vi "wd_replaceInIndexFindNext.vi"(9 "Next in":i32, 10 "LengthIn":u64, 11 "RecordInfo":T1[](array[typedef])) -> (2 "LengthOut":u64, 3 "Next out":i32)   [LabVIEW 2020, in "NI_ExcelFile.lvlib"]
uses:
  <vilib>/express/express shared/NI_ExcelFile/NI_ExcelFile.lvlib
  <vilib>/express/express shared/NI_ExcelFile/Ctrls/wd_recordInfo.ctl
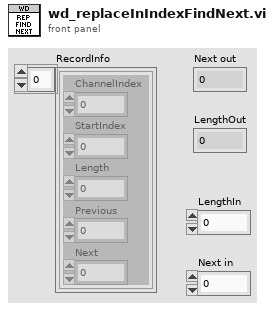
[diagram p1: front panel]
types:
  T1 = typedef "NI_ExcelFile.lvlib/wd_recordInfo.ctl" = cluster{"ChannelIndex":u32, "StartIndex":u64, "Length":u64, "Previous":i32, "Next":i32}
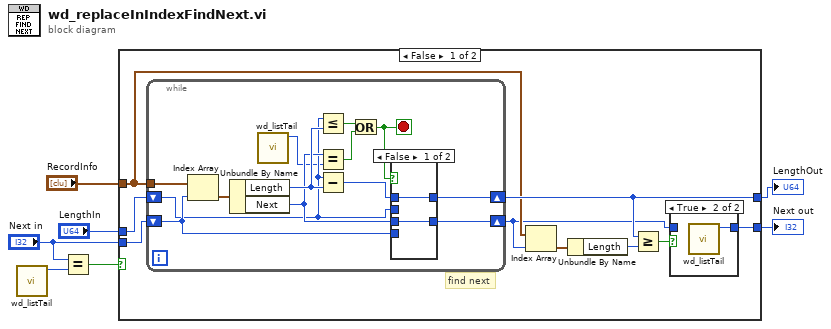
[diagram p0: block diagram]
diagram:
  n1 = call <vilib>:"wd_listTail.vi"() -> ("list tail"=w1:i32)  [unwired: 11 in]
  n2 = Equal?(x="Next in", y=w1) -> (x = y?=w7:bool)
  n3 = case shown="False" w7 {
    tunnel: "LengthIn" -> [w16 w37]
    tunnel: [w15 w37] -> w3
    tunnel: "RecordInfo" -> [w14 _]
    tunnel: [w9 w36] -> w5
    tunnel: "Next in" -> [w8 w36]
    frame False {
      # "find next"
      n4 = while {
        shift-right: [w21] -> w15
        shift-left: w16 -> [w22]
        tunnel: w14 -> [w29]
        shift-right: [w25] -> w10
        shift-left: w8 -> [w23]
        stop <- w26 stop-if-true
        n5 = Index Array(array=w29, index=w23) -> (element=w31:T1)
        n6 = Unbundle By Name(w31) -> ("Length"=w30:u64, "Next"=w24:i32)
        n7 = call <vilib>:"wd_listTail.vi"() -> ("list tail"=w19:i32)  [unwired: 11 in]
        n8 = Less Or Equal?(x=w22, y=w30) -> (x <= y?=w28:bool)
        n9 = Equal?(x=w24, y=w19) -> (x = y?=w27:bool)
        n10 = Subtract(x=w22, y=w30) -> (x-y=w20:u64)
        n11 = Or(x=w28, y=w27) -> (x .or. y?=w26:bool)
        n12 = case shown="False" w26 {
          tunnel: [w33 w35] -> w25
          tunnel: w24 -> [w33 _]
          tunnel: w23 -> [_ w35]
          tunnel: w22 -> [_ w34]
          tunnel: [w32 w34] -> w21
          tunnel: w20 -> [w32 _]
          frame False {
          }
          frame True {
          }
        }
      }
      n13 = Index Array(array=w14, index=w10) -> (element=w13:T1)
      n14 = Unbundle By Name(w13) -> ("Length"=w12:u64)
      n15 = Greater Or Equal?(x=w15, y=w12) -> (x >= y?=w11:bool)
      n16 = case shown="True" w11 {
        tunnel: [w17 w18] -> w9
        tunnel: w10 -> [w17 _]
        frame False {
        }
        frame True {
          n17 = call <vilib>:"wd_listTail.vi"() -> ("list tail"=w18:i32)  [unwired: 11 in]
        }
      }
    }
    frame True {
    }
  }
  "Next out" <- w5
  "LengthOut" <- w3
